vi "error.To JSON String.vi"(8 "error in (no error)":errorcluster, 11 "error in":refnum<class "error.lvclass">) -> (0 "error out":errorcluster, 2 "JSON String":string, 3 "error out":refnum<class "error.lvclass">)   [LabVIEW 2020, in "JSON-RPC Lib.lvlib" / "error.lvclass"]
uses:
  error.lvclass
  Variant JSON API/Variant JSON API.lvlib
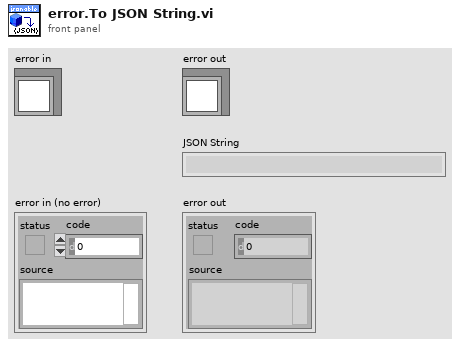
[diagram p1: front panel]
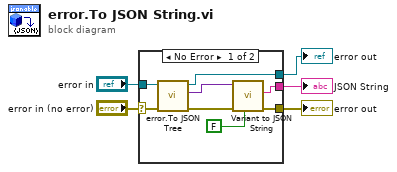
[diagram p0: block diagram]
diagram:
  n1 = case shown="No Error" "error in (no error)" {
    selector: "error in (no error)" -> [w12 w15]
    tunnel: [w8 w15] -> w4
    tunnel: [w11 w14] -> w2
    tunnel: "error in" -> [w13 w14]
    tunnel: [w9 _] -> w1
    frame No Error {
      n2 = call "error.To JSON Tree.vi"("error in (no error)"=w12, "error in"=w13) -> (0:"error out"=w7:errorcluster, "JSON Value out"=w10:variant, 3:"error out"=w11:refnum<class "error.lvclass">)  [unwired: 7 in]
      n3 = call "Variant to JSON String.vi"("pretty print? (F)"=FALSE ("pretty print? (T)"), "error in (no error)"=w7, "Variant in"=w10) -> ("error out"=w8:errorcluster, "String"=w9:string)  [unwired: 6 in, 1 out]
    }
    frame Error {
    }
  }
  "error out" <- w4
  "error out" <- w2
  "JSON String" <- w1
